vi "Set Target Field.vi"(2 "error in":T1, 3 "Target Field (kG)":dbl format="%.3f", 4 "VISA resource name":refnum<visa-resource-name>) -> (0 "error out":T1, 1 "VISA resource name out":refnum<visa-resource-name>)   [LabVIEW 2019]
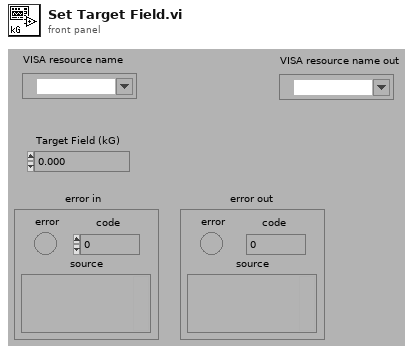
[diagram p1: front panel]
types:
  T1 = cluster{"error":bool, "code":i32, "source":string}
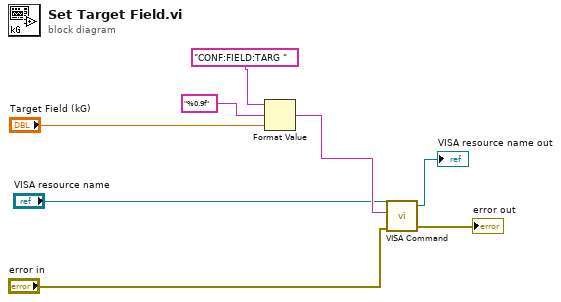
[diagram p0: block diagram]
diagram:
  n1 = Format Value(string ("")="CONF:FIELD:TARG ", format string="%0.9f", value (0)="Target Field (kG)") -> (output string=w4:string)
  n2 = call "VISA Command.vi"("error in (no error)"="error in", "Command"=w4, "VISA resource name"="VISA resource name") -> ("error out"=→"error out":errorcluster, "VISA resource name out"=→"VISA resource name out":refnum<visa-resource-name>)  [unwired: 1 in, 1 out]
